vi "Cairo.GetSUVDataFromFile.vi"(8 "Error In":errorcluster, 9 "TestNumbers":string[](array[string]), 10 "SerialNumber":string, 11 "Refnum":T1) -> (0 "Error Out":errorcluster, 2 "Data Out":dbl[](array[numeric]))   [LabVIEW 2019]
uses:
  <vilib>/Utility/config.llb/Config Data RefNum.ctl
  <vilib>/Utility/config.llb/Read Key (Double).vi
  <vilib>/Utility/config.llb/NI_LVConfig.lvlib
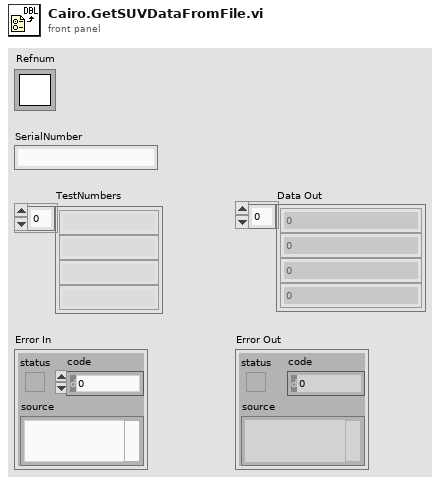
[diagram p1: front panel]
types:
  T1 = typedef "NI_LVConfig.lvlib/Config Data RefNum.ctl" = refnum<k1>
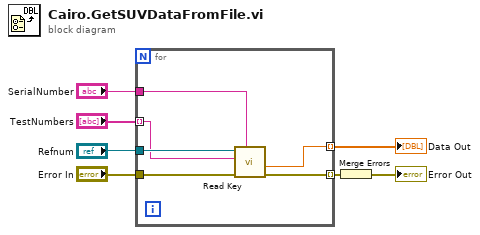
[diagram p0: block diagram]
diagram:
  n1 = for {
    tunnel: "Refnum" -> [w13]
    tunnel: "Error In" -> [w12]
    tunnel: [w11] -> w4 mode=indexing
    tunnel: [w10] -> w5 mode=indexing
    tunnel: "SerialNumber" -> [w9]
    tunnel: "TestNumbers" -> [w8] mode=indexing
    n2 = call-poly <vilib>:"Read Key.vi"("section"=w9, "error in (no error)"=w12, "key"=w8, "refnum"=w13) -> ("error out"=w11:errorcluster, "value"=w10:dbl)  [unwired: 4 in, 2 out]
  }
  "Data Out" <- w5
  n3 = Merge Errors(w4) -> (→"Error Out":errorcluster)
